vi "Example-Waveform Circular Buffer.vi"() -> ()   [LabVIEW 2019]
uses:
  <vilib>/measure/NI_MABase.lvlib
panel:
  out "Acquired Segment":waveform(dbl)(graph)={"t0"=timestamp(321.0 s since 1904-01-01), "dt"=0.001, "Y"=array[1000 elements]}
  in  "square wave amplitude":dbl(knob) scale=-4.0..4.0
  in  "buffer duration (s)":dbl=10.0
  out "Acquisition History":waveform(dbl)(graph)={"t0"=timestamp(311.0 s since 1904-01-01), "dt"=0.001, "Y"=array[10000 elements]}
  in  "stop":bool
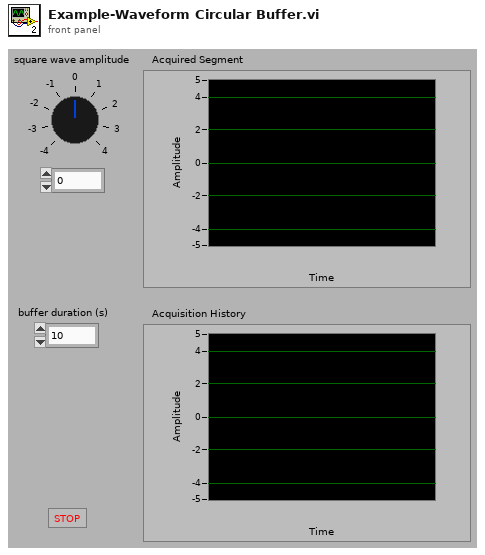
[diagram p1: front panel]
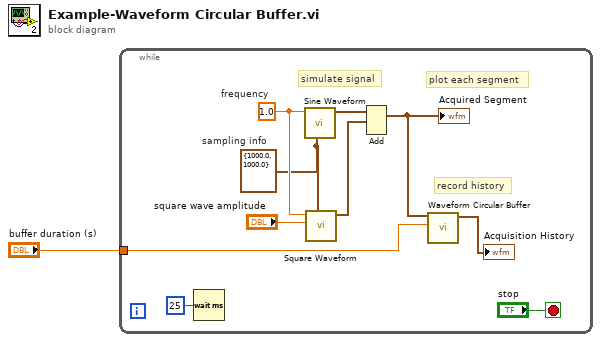
[diagram p0: block diagram]
diagram:
  n1 = while {
    tunnel: "buffer duration (s)" -> [w7]
    stop <- "stop" stop-if-true
    w3 = cluster{"Fs":dbl, "#s":dbl} {"Fs"=1000.0, "#s"=1000.0}  # sampling info
    w11 = 1.0  # frequency
    # "plot each segment"
    # "record history"
    # "simulate signal"
    n2 = Wait (ms)(milliseconds to wait=u32 25) -> ()  [unwired: 1 out]
    n3 = call <vilib>:"Sine Waveform.vi"("sampling info"=w3, "frequency"=w11) -> ("signal out"=w10:waveform(dbl))  [unwired: 8 in, 1 out]
    n4 = call <vilib>:"Square Waveform.vi"("sampling info"=w3, "amplitude"="square wave amplitude", "frequency"=w11) -> ("signal out"=w9:waveform(dbl))  [unwired: 7 in, 1 out]
    n5 = Add(1:w9, 2:w10) -> (0:w2:waveform(dbl))  [unwired: 1 in, 1 out]
    "Acquired Segment" <- w2
    n6 = call "Waveform Circular Buffer.vi"("buffer duration (s)"=w7, "waveform in"=w2) -> ("waveform out"=→"Acquisition History":waveform(dbl))  [unwired: 8 in, 1 out]
  }
